vi "ge_ColInfo.vi"(8 "error in":errorcluster, 10 "Active Cell":T4, 11 "Table Ref":refnum<vi>) -> (0 "error out":errorcluster, 2 "Ctrl Size Pos":T3)   [LabVIEW 2018]
uses:
  <vilib>/Utility/miscctls.llb/LVRowAndColumnTypeDef.ctl
  <vilib>/Utility/miscctls.llb/LVPositionTypeDef.ctl
  <vilib>/Utility/miscctls.llb/LVBoundsTypeDef.ctl
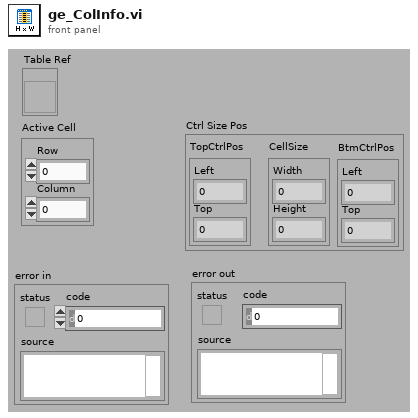
[diagram p1: front panel]
types:
  T1 = typedef "LVPositionTypeDef.ctl" = cluster{"Left":i32, "Top":i32}
  T2 = typedef "LVBoundsTypeDef.ctl" = cluster{"Width":u32, "Height":u32}
  T3 = cluster{"TopCtrlPos":T1, "CellSize":T2, "BtmCtrlPos":T1}
  T4 = typedef "LVRowAndColumnTypeDef.ctl" = cluster{"Row":i32, "Column":i32}
  T5 = cluster{"ActiveCellPos":T1, "CellSize":T2, "ActiveCellPos":T1}
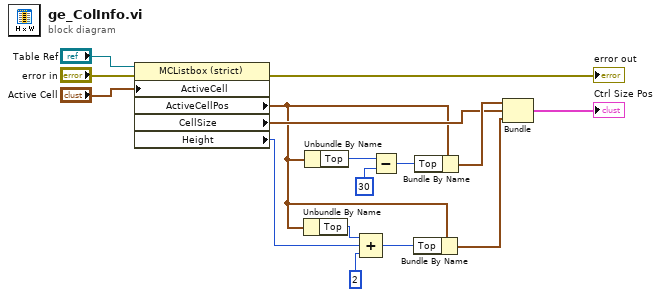
[diagram p0: block diagram]
diagram:
  n1 = property on="Property Node" class="MCListbox (strict)"(reference="Table Ref", error in="error in", "ActiveCell"="Active Cell") -> (error out=→"error out":errorcluster, "ActiveCellPos"=w5:T1, "CellSize"=w12:T2, "Height"=w3:u32)  [unwired: 1 out]
  n2 = Unbundle By Name(w5) -> ("Top"=w4:i32)
  n3 = Unbundle By Name(w5) -> ("Top"=w16:i32)
  n4 = Compound Arithmetic op=ADD(w4, w3, u32 2 ("value")) -> (w2:u32)
  n5 = Subtract(x=w16, y=30) -> (x-y=w14:i32)
  n6 = Bundle By Name(cluster=w5, "Top"=w2) -> (w6:T1)
  n7 = Bundle By Name(cluster=w5, "Top"=w14) -> (w13:T1)
  n8 = Bundle("ActiveCellPos"=w13, "CellSize"=w12, "ActiveCellPos"=w6) -> (→"Ctrl Size Pos":T5)  [unwired: 1 in]
